vi "Stop Big Deltas.vi"(3 "Right Grabber Requested Position":dbl, 4 "Method of Calc Good Pos":T1(ring), 5 "Left Grabber Requested Position":dbl) -> (0 "Experimental Left Grabber Good Position":dbl, 1 "Experimental Right Grabber Good Position":dbl, 2 "Is Big Delta?":bool)   [LabVIEW 2015]
uses:
  Global Variables/Settings.vi
  Global Variables/refnum names.vi
panel:
  out "Percent off":dbl
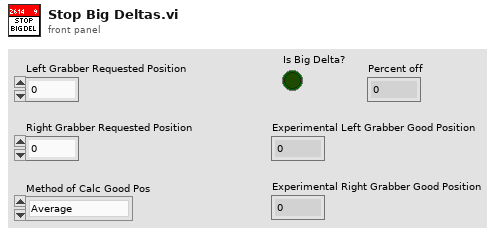
[diagram p1: front panel]
types:
  T1 = enum16{"Average", "Use Left Grabber", "Use Right Grabber", "Stop (Use Current Position)", "Passthrough"}
  T2 = typedef "WPI_MotorControlDeviceRef.ctl" = cluster{"DeviceStatus":errorcluster, "Type":T3, "PWM":cluster{"PWM Channel":T4, "DeadBand":T5}, "CAN":cluster{"Device Number":u8, "Control Mode":T6, "Semaphore":T7, "Max Vout":dbl, "TalonSRX Control Mode":T8}, "Invert":bool}
  T3 = typedef "WPI_MotorControlType.ctl" = enum16{"PWM", "CAN", "CANTalonSRX"}
  T4 = typedef "FPGA_DIOPWMChannel.ctl" = enum8{"PWM 0", "PWM 1", "PWM 2", "PWM 3", "PWM 4", "PWM 5", "PWM 6", "PWM 7", "PWM 8", "PWM 9", "PWM MXP 0", "PWM MXP 1", "PWM MXP 2", "PWM MXP 3", "PWM MXP 4", "PWM MXP 5", "PWM MXP 6", "PWM MXP 7", "PWM MXP 8", "PWM MXP 9", "Invalid"}
  T5 = typedef "WPI_PWMDeadband.ctl" = cluster{"Name":string, "maxPositivePwm":i32, "minPositivePwm":i32, "centerPwm":i32, "maxNegativePwm":i32, "minNegativePwm":i32, "angularRange":u16}
  T6 = typedef "WPI_CANJaguar_ControlMode.ctl" = enum8{"Percent VBus", "Current", "Speed", "Position", "Voltage"}
  T7 = typedef "Semaphore RefNum" = refnum<k1>
  T8 = typedef "WPI_CANTalonSRX_APIControlMode.ctl" = enum8{"Percent VBus", "Speed", "Position", "Slave", "Unchanged / Invalid", "Voltage Compensation", "Current", "Motion Profile"}
  T9 = typedef "WPI_CANTalonSRX_GlobalStatus.ctl" = cluster{"Applied Throttle":dbl, "Module Enabled":bool, "CAN Error":errorcluster, "Closed Loop Error":dbl, "Forward Limit Switch Closed":bool, "Reverse Limit Switch Closed":bool, "Sensor Position":dbl, "Sensor Velocity":dbl, "Current":dbl, "Sticky Fault - Over Temp":bool, "Sticky Fault - Under Voltage":bool, "Sticky Fault - Forward Limit":bool, "Sticky Fault - Reverse Limit":bool, "Sticky Fault - Forward Soft Limit":bool, "Sticky Fault - Reverse Soft Limit":bool, "Brake is Enabled":bool, "Encoder Position":dbl, "Encoder Velocity":dbl, "Encoder Index Count":dbl, "Encoder A Pin State":bool, "Encoder B Pin State":bool, "Encoder Index Pin State":bool, "Analog In":dbl, "Analog In Velocity":dbl, "Temperature (C)":dbl, "Battery Voltage":dbl, "Control 5 Is Supported":bool, "Current Profile Slot Select":dbl, "Pos Div 8":bool, "Vel Div 4":bool, "Pulse Width Position":i32, "Pulse Width Velocity":i32, "Pulse Width Rise To Rise (us)":i32, "Pulse Width Rise To Fall (us)":i32, "Mot Prof Active Is Under Run":bool, "Mot Prof Active Has Under Run":bool, "Mot Prof Active Is Last":bool, "Mot Prof Active Velocity Only":bool, "Mot Prof Active Is Valid":bool, "Mot Prof Buffer Is Full":bool, "Mot Prof Active Profile Slot Select":i32, "Mot Prof NextID":i32, "Mot Prof Count":i32, "Mot Prof Active Velocity":dbl, "Mot Prof Active Position":dbl, "Mot Prof Output Enable":i32}
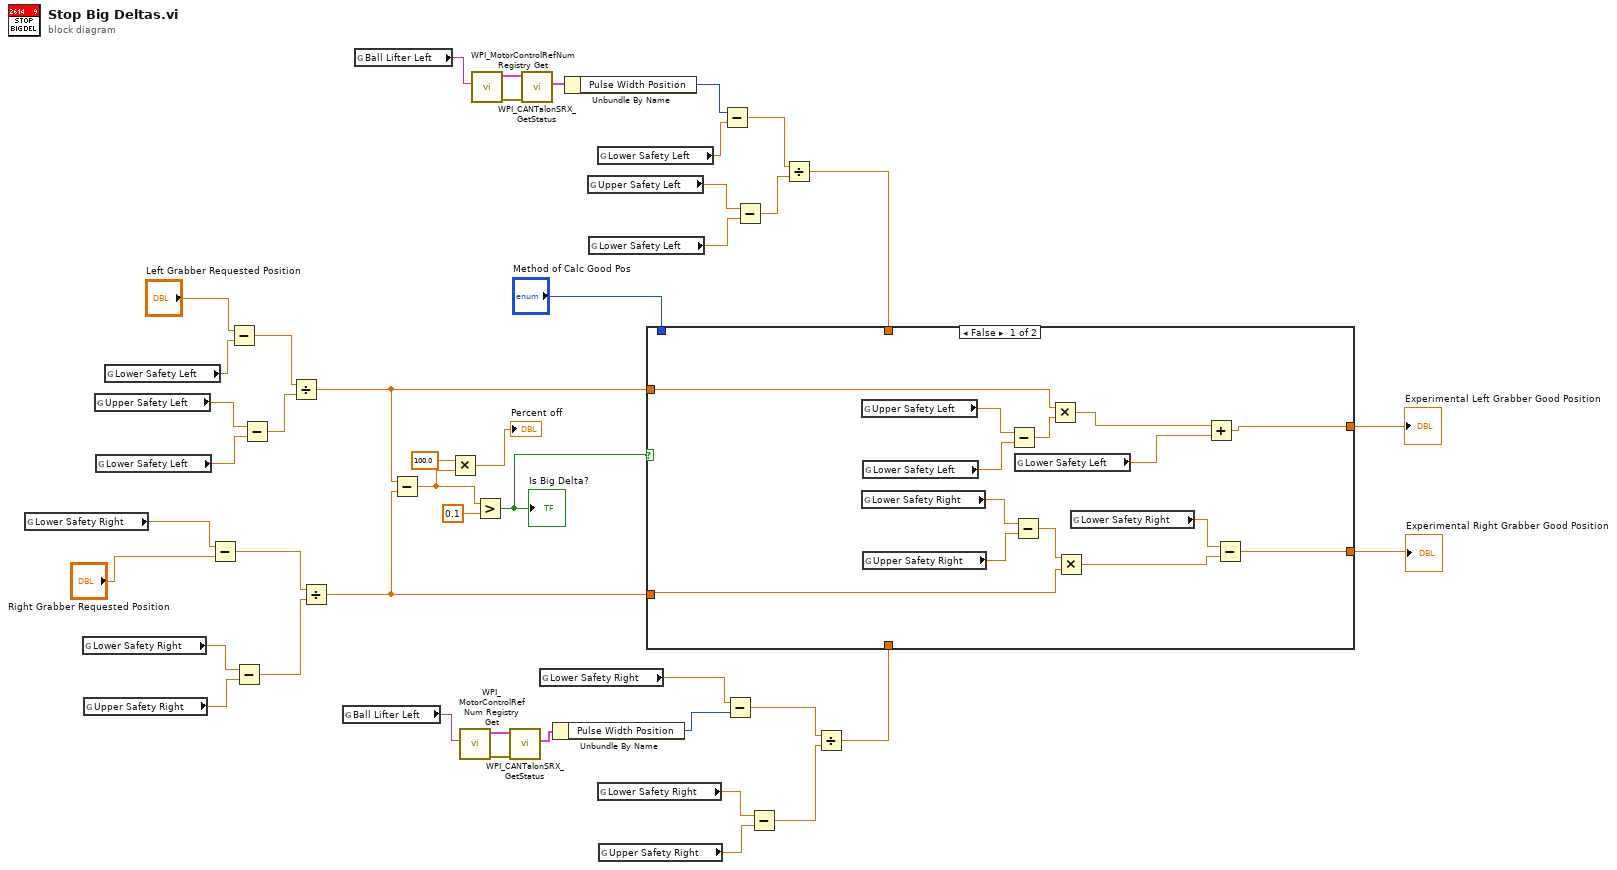
[diagram p0: block diagram]
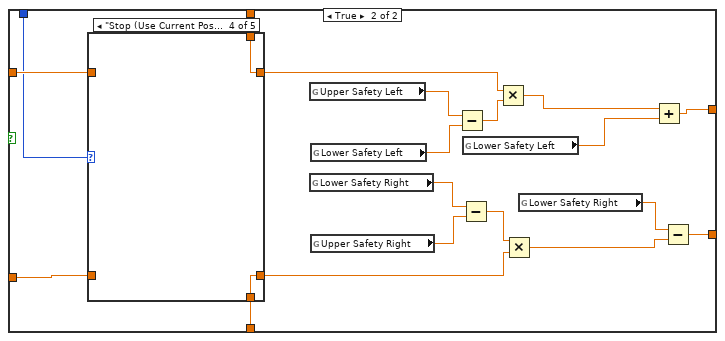
[diagram p2: hidden frame]
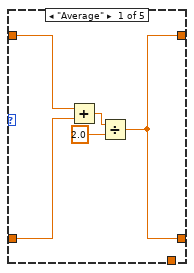
[diagram p3: hidden frame]
diagram:
  n1 = global read "Settings.vi" "Lower Safety Right"() -> (w33:dbl)
  n2 = global read "Settings.vi" "Lower Safety Right"() -> (w40:dbl)
  n3 = global read "Settings.vi" "Upper Safety Right"() -> (w41:dbl)
  n4 = global read "Settings.vi" "Upper Safety Left"() -> (w44:dbl)
  n5 = global read "Settings.vi" "Lower Safety Left"() -> (w43:dbl)
  n6 = global read "Settings.vi" "Lower Safety Left"() -> (w36:dbl)
  n7 = Subtract(x=w33, y="Right Grabber Requested Position") -> (x-y=w35:dbl)
  n8 = Subtract(x="Left Grabber Requested Position", y=w36) -> (x-y=w38:dbl)
  n9 = Subtract(x=w40, y=w41) -> (x-y=w39:dbl)
  n10 = Subtract(x=w44, y=w43) -> (x-y=w42:dbl)
  n11 = Divide(x=w38, y=w42) -> (x/y=w29:dbl)
  n12 = Divide(x=w35, y=w39) -> (x/y=w30:dbl)
  n13 = global read "refnum names.vi" "Ball Lifter Left"() -> (w8:string)
  n14 = global read "refnum names.vi" "Ball Lifter Left"() -> (w1:string)
  n15 = Subtract(x=w29, y=w30) -> (x-y=w11:dbl)
  n16 = Multiply(x=100.0, y=w11) -> (x*y=→"Percent off":dbl)
  n17 = call <vilib>:"WPI_MotorControlRefNum Registry Get.vi"("refnum name"=w8) -> ("error out"=w5:errorcluster, "MotorControlDevRef"=w6:T2)  [unwired: 9 in]
  n18 = call <vilib>:"WPI_MotorControlRefNum Registry Get.vi"("refnum name"=w1) -> ("error out"=w4:errorcluster, "MotorControlDevRef"=w3:T2)  [unwired: 9 in]
  n19 = Greater?(x=w11, y=0.1) -> (0:w31:bool)
  "Is Big Delta?" <- w31
  n20 = call <vilib>:"WPI_CANTalonSRX_GetStatus.vi"("error in (no error)"=w5, "CAN Talon SRX Ref"=w6) -> ("Talon SRX Status"=w7:T9)  [unwired: 7 in, 2 out]
  n21 = call <vilib>:"WPI_CANTalonSRX_GetStatus.vi"("error in (no error)"=w4, "CAN Talon SRX Ref"=w3) -> ("Talon SRX Status"=w2:T9)  [unwired: 7 in, 2 out]
  n22 = global read "Settings.vi" "Lower Safety Right"() -> (w21:dbl)
  n23 = Unbundle By Name(w7) -> ("Pulse Width Position"=w16:i32)
  n24 = Unbundle By Name(w2) -> ("Pulse Width Position"=w22:i32)
  n25 = global read "Settings.vi" "Upper Safety Left"() -> (w23:dbl)
  n26 = global read "Settings.vi" "Lower Safety Left"() -> (w24:dbl)
  n27 = global read "Settings.vi" "Lower Safety Left"() -> (w27:dbl)
  n28 = global read "Settings.vi" "Lower Safety Right"() -> (w18:dbl)
  n29 = global read "Settings.vi" "Upper Safety Right"() -> (w17:dbl)
  n30 = Subtract(x=w22, y=w27) -> (x-y=w26:dbl)
  n31 = Subtract(x=w21, y=w16) -> (x-y=w20:dbl)
  n32 = Subtract(x=w23, y=w24) -> (x-y=w25:dbl)
  n33 = Subtract(x=w18, y=w17) -> (x-y=w19:dbl)
  n34 = Divide(x=w26, y=w25) -> (x/y=w14:dbl)
  n35 = Divide(x=w20, y=w19) -> (x/y=w15:dbl)
  n36 = case shown="False" w31 {
    tunnel: w30 -> [w47 w76]
    tunnel: w29 -> [w48 w77]
    tunnel: "Method of Calc Good Pos" -> [_ w75]
    tunnel: w15 -> [_ w74]
    tunnel: w14 -> [_ w73]
    tunnel: [w45 w60] -> w13
    tunnel: [w46 w59] -> w12
    frame False {
      n37 = global read "Settings.vi" "Upper Safety Left"() -> (w57:dbl)
      n38 = global read "Settings.vi" "Lower Safety Right"() -> (w53:dbl)
      n39 = global read "Settings.vi" "Lower Safety Left"() -> (w58:dbl)
      n40 = global read "Settings.vi" "Upper Safety Right"() -> (w52:dbl)
      n41 = Subtract(x=w57, y=w58) -> (x-y=w56:dbl)
      n42 = Subtract(x=w53, y=w52) -> (x-y=w51:dbl)
      n43 = global read "Settings.vi" "Lower Safety Left"() -> (w54:dbl)
      n44 = Multiply(x=w48, y=w56) -> (x*y=w55:dbl)
      n45 = Multiply(x=w51, y=w47) -> (x*y=w50:dbl)
      n46 = global read "Settings.vi" "Lower Safety Right"() -> (w49:dbl)
      n47 = Add(x=w55, y=w54) -> (x+y=w45:dbl)
      n48 = Subtract(x=w49, y=w50) -> (x-y=w46:dbl)
    }
    frame True {
      n49 = case shown="\"Stop (Use Current Position)\"" w75 {
        tunnel: w77 -> [w78 w83 _ _ w88]
        tunnel: w76 -> [w81 _ w84 _ w87]
        tunnel: [w79 w83 w84 w85 w88] -> w69
        tunnel: [w79 w83 w84 w86 w87] -> w64
        tunnel: w74 -> [_ _ _ w86 _]
        tunnel: w73 -> [_ _ _ w85 _]
        frame "Average" {
          n50 = Add(x=w78, y=w81) -> (x+y=w82:dbl)
          n51 = Divide(x=w82, y=2.0) -> (x/y=w79:dbl)
        }
        frame "Use Left Grabber" {
        }
        frame "Use Right Grabber" {
        }
        frame "Stop (Use Current Position)" {
        }
        frame "Passthrough" {
        }
      }
      n52 = global read "Settings.vi" "Upper Safety Left"() -> (w71:dbl)
      n53 = global read "Settings.vi" "Lower Safety Right"() -> (w66:dbl)
      n54 = global read "Settings.vi" "Lower Safety Left"() -> (w72:dbl)
      n55 = global read "Settings.vi" "Upper Safety Right"() -> (w65:dbl)
      n56 = Subtract(x=w71, y=w72) -> (x-y=w70:dbl)
      n57 = Subtract(x=w66, y=w65) -> (x-y=w63:dbl)
      n58 = global read "Settings.vi" "Lower Safety Left"() -> (w67:dbl)
      n59 = Multiply(x=w69, y=w70) -> (x*y=w68:dbl)
      n60 = Multiply(x=w63, y=w64) -> (x*y=w62:dbl)
      n61 = global read "Settings.vi" "Lower Safety Right"() -> (w61:dbl)
      n62 = Add(x=w68, y=w67) -> (x+y=w60:dbl)
      n63 = Subtract(x=w61, y=w62) -> (x-y=w59:dbl)
    }
  }
  "Experimental Left Grabber Good Position" <- w13
  "Experimental Right Grabber Good Position" <- w12
